vi "Program24.vi"() -> ()   [LabVIEW 2020]
panel:
  in  "Cluster":T1
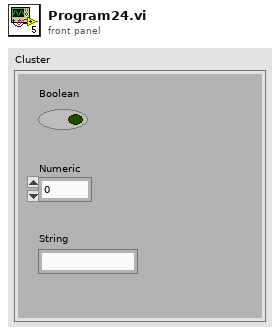
[diagram p1: front panel]
types:
  T1 = cluster{"Boolean":bool, "Numeric":dbl, "String":string}
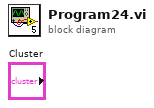
[diagram p0: block diagram]
diagram:
